vi "subSetItemInfoDependencies.vi"(8 "error in (no error)":errorcluster, 11 "SolutionBuilder in":refnum<class "SolutionBuilder.lvclass">) -> (0 "error out":errorcluster, 3 "SolutionBuilder out":refnum<class "SolutionBuilder.lvclass">)   [LabVIEW 2019, in "SolutionBuilder.lvlib" / "SolutionBuilder.lvclass"]
uses:
  SolutionBuilder.lvclass
  ProjectItem/ProjectItem.lvclass
  NamePathMap.ctl
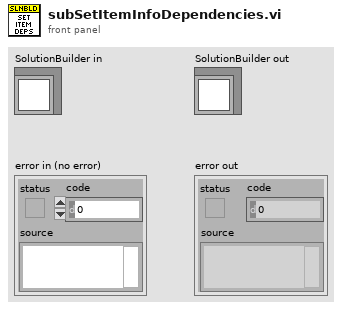
[diagram p1: front panel]
types:
  T1 = typedef "SolutionBuilder.lvlib/SolutionBuilder.lvclass/NamePathMap.ctl" = map{string, path}
  T2 = typedef "SolutionBuilder.lvlib/SolutionBuilder.lvclass/ProjectItemMap.ctl" = map{path, refnum<class "ProjectItem.lvclass">[]}
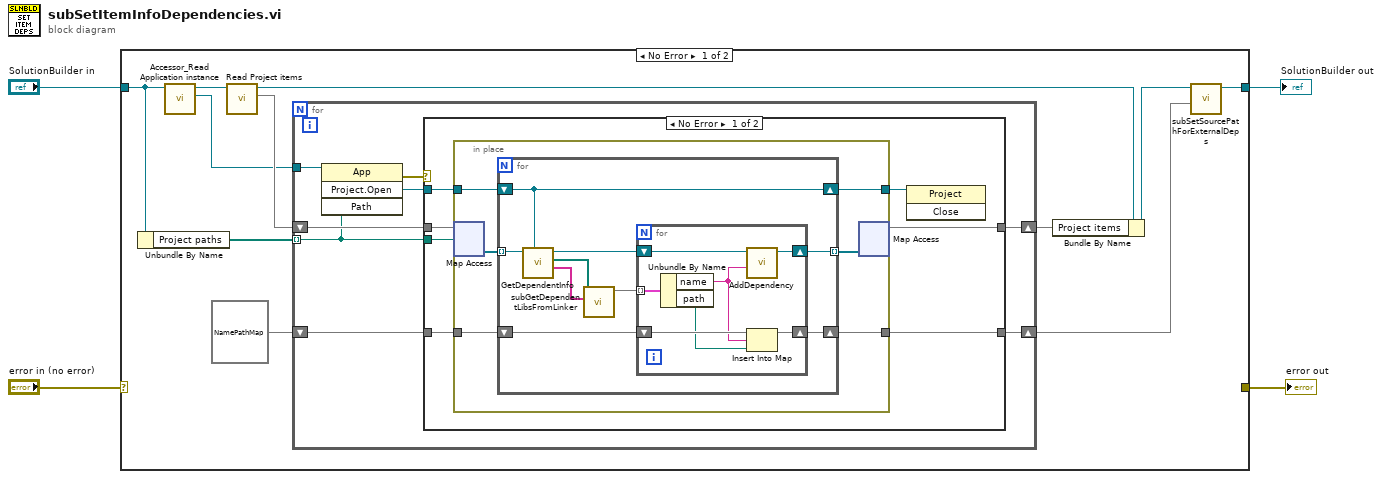
[diagram p0: block diagram]
diagram:
  n1 = case shown="No Error" "error in (no error)" {
    selector: "error in (no error)" -> [_ w55]
    tunnel: [w9 w56] -> w4
    tunnel: "SolutionBuilder in" -> [w8 w56]
    tunnel: [_ w55] -> w1
    frame No Error {
      n2 = Unbundle By Name(w8) -> ("Project paths"=w15:path[])
      n3 = call "Accessor_Read Application instance.vi"("SolutionBuilder in"=w8) -> ("App instance"=w6:refnum<vi>, "SolutionBuilder out"=w7:refnum<class "SolutionBuilder.lvclass">)  [unwired: 8 in, 1 out]
      n4 = call-dynamic "Read Project items.vi"("SolutionBuilder in"=w7) -> ("Project items"=w14:T2, "SolutionBuilder out"=w13:refnum<class "SolutionBuilder.lvclass">)  [unwired: 9 in]
      n5 = for {
        tunnel: w15 -> [w19] mode=indexing
        shift-right: [w22] -> w12
        shift-left: w14 -> [w23]
        shift-right: [w20] -> w11
        shift-left: T1 {} ("Dependency libs") -> [w21]
        tunnel: w6 -> [w18]
        n6 = invoke class="App" method="Project.Open"(reference=w18, "Path"=w19) -> (error out=w17:errorcluster, "Project:Open"=w16:refnum<vi>)  [unwired: 2 in, 2 out]
        n7 = case shown="No Error" w17 {
          tunnel: w23 -> [w30 w54]
          tunnel: [w29 w54] -> w22
          tunnel: w21 -> [w28 w53]
          tunnel: [w27 w53] -> w20
          tunnel: w19 -> [w26 _]
          tunnel: w16 -> [w25 _]
          frame No Error {
            n8 = in-place {
              in-place-border: [w34] -> w27
              in-place-border: w28 -> [w33]
              in-place-border: w25 -> [w32]
              in-place-border: [w31] -> w24
              n9 = in-place-map #1(w30, w26) -> (w36:refnum<class "ProjectItem.lvclass">[])  [unwired: 1 in, 1 out]
              n10 = for {
                tunnel: w36 -> [w40] mode=indexing
                tunnel: [w45] -> w35 mode=indexing
                shift-right: [w44] -> w34
                shift-left: w33 -> [w43]
                shift-right: [w41] -> w31
                shift-left: w32 -> [w41]
                n11 = call "GetDependentInfo.vi"("Project ref"=w41, "ProjectItem in"=w40) -> ("Dependent owning libs"=w37:string[], "Dependent paths"=w38:path[], "ProjectItem out"=w39:refnum<class "ProjectItem.lvclass">)  [unwired: 6 in, 1 out]
                n12 = call "subGetDependentLibsFromLinker.vi"("Owning libs"=w37, "Paths"=w38) -> ("Dependency libs"=w42:T1)  [unwired: 9 in]
                n13 = for {
                  tunnel: w42 -> [w48] mode=indexing
                  shift-right: [w51] -> w45
                  shift-left: w39 -> [w52]
                  shift-right: [w50] -> w44
                  shift-left: w43 -> [w49]
                  n14 = Unbundle By Name(w48) -> ("name"=w47:string, "path"=w46:path)
                  n15 = call-dynamic "AddDependency.vi"("Dependency"=w47, "ProjectItem in"=w52) -> ("ProjectItem out"=w51:refnum<class "ProjectItem.lvclass">)  [unwired: 8 in, 1 out]
                  n16 = Insert Into Map(map in=w49, key=w47, value=w46) -> (map out=w50:T1)  [unwired: 2 out]
                }
              }
              n17 = in-place-map #1(w35) -> (w29:T2)  [unwired: 1 in, 2 out]
            }
            n18 = invoke class="Project" method="Close"(reference=w24) -> ()  [unwired: 2 in, 3 out]
          }
          frame Error {
          }
        }
      }
      n19 = Bundle By Name(cluster=w13, "Project items"=w12) -> (w10:refnum<class "SolutionBuilder.lvclass">)
      n20 = call "subSetSourcePathForExternalDeps.vi"("Dependency libs"=w11, "SolutionBuilder in"=w10) -> ("SolutionBuilder out"=w9:refnum<class "SolutionBuilder.lvclass">)  [unwired: 8 in, 1 out]
    }
    frame Error {
    }
  }
  "SolutionBuilder out" <- w4
  "error out" <- w1
